vi "EOL CAN_Get_Motor_Temperature.vi"(11 "NetworkObjHandle":u32) -> (1 "Motor Temperature":dbl, 2 "TxRx Data":string[][](array[string]), 3 "Response Good?":bool)   [LabVIEW 2012]
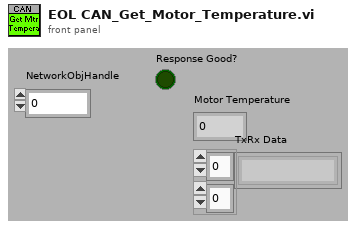
[diagram p1: front panel]
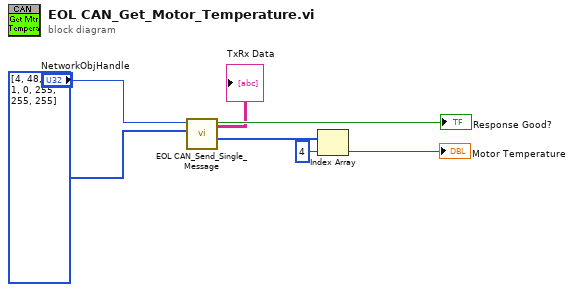
[diagram p0: block diagram]
diagram:
  n1 = call "EOL CAN_Send_Single_Message.vi"("Read Session in"=u8[] [4, 48, 18, 1, 0, 255, 255, 255] ("Transmit Data"), "Write Session in"="NetworkObjHandle") -> ("Rx Message"=w4:u8[], "Response Good?"=→"Response Good?":bool, "TxRx Data"=→"TxRx Data":string[][])  [unwired: 5 in, 2 out]
  n2 = Index Array(array=w4, index=4) -> (element=→"Motor Temperature":u8)
